vi "Initialise devices.vi"() -> (5 "Number of connected devices":u32, 6 "Device handles":u32[](array[numeric]), 7 "Laser comms. error":errorcluster[](array[cluster]), 8 "Get lasers serial num. error":errorcluster, 9 "Device detection error":errorcluster, 10 "Device initialisation errors":errorcluster[](array[cluster]))   [LabVIEW 2014]
uses:
  Commands.ctl
  Coherent global.vi
panel:
  # "PN 05/11/2014"
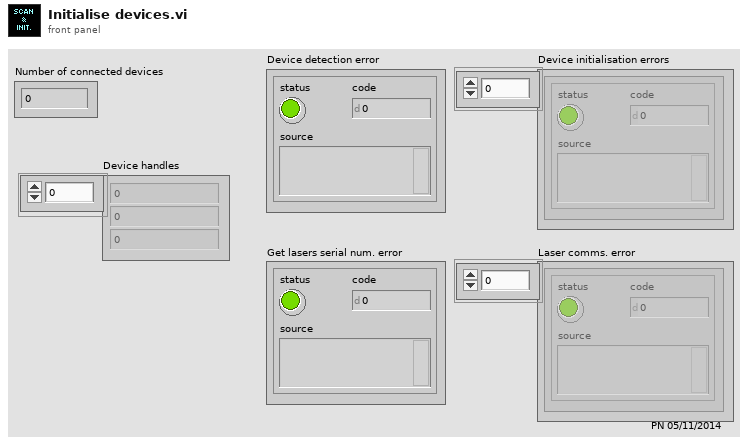
[diagram p1: front panel]
types:
  T1 = typedef "Commands.ctl" = u8
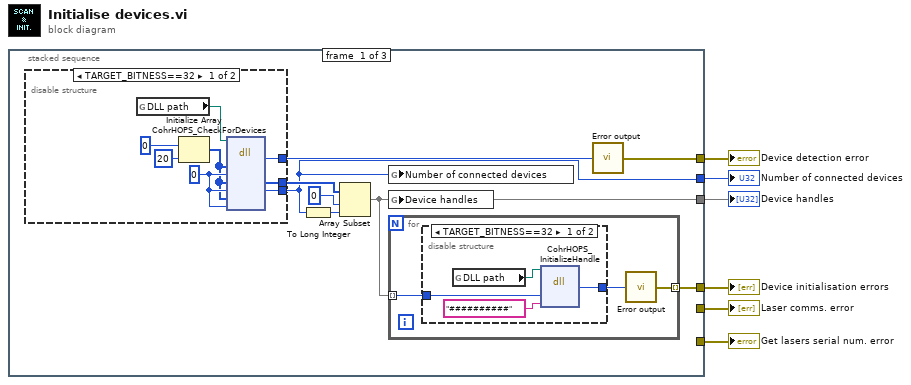
[diagram p0: block diagram]
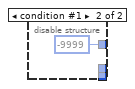
[diagram p2: hidden frame]
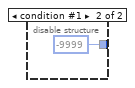
[diagram p3: hidden frame]
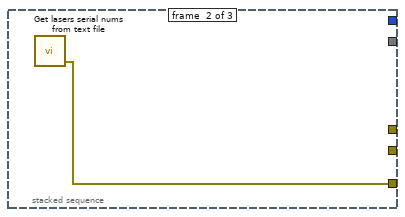
[diagram p4: hidden frame]
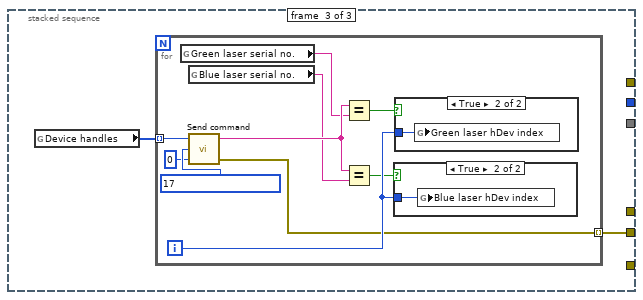
[diagram p5: hidden frame]
diagram:
  n1 = stacked-sequence {
    tunnel: [w11 _ _] -> w6
    tunnel: [w10 _ _] -> w5
    tunnel: [w9 _ _] -> w4
    tunnel: [w7 _ _] -> w3
    tunnel: [_ w32 _] -> w2
    tunnel: [_ _ w33] -> w1
    frame #0 {
      n2 = disable-structure shown="TARGET_BITNESS==32" {
        disable-tunnel: [w18 -9999 ("return value")] -> w12
        disable-tunnel: [w17 _] -> w8
        disable-tunnel: [w16 _] -> w7
        frame condition #0 (active) {
          w22 = u32 0 ("Input Value")
          n3 = global read "Coherent global.vi" "DLL path"() -> (w15:path)
          n4 = Initialize Array(u32 0 ("Input Value"), 20 ("dimension size")) -> (w19:u32[])
          n5 = dll-call lib="C:/Program Files (x86)/Coherent/HOPS/CohrHOPS.dll" fn="CohrHOPS_CheckForDevices"(path in=w15, "devicesConnected"=w19, "numberOfDevicesConnected"=w22, "devicesAdded"=w19, "numberOfDevicesAdded"=w22, "devicesRemoved"=w19, "numberOfDevicesRemoved"=w22) -> ("return value"=w18:i32, "devicesAdded"=w17:u32[], "numberOfDevicesAdded"=w16:u32)  [unwired: 6 in, 2 out]
        }
        frame condition #1 {
        }
      }
      n6 = To Long Integer(number=w7) -> (32bit integer=w14:i32)
      n7 = Array Subset(array=w8, index=0, length=w14) -> (w11:u32[])
      n8 = global write "Coherent global.vi" "Number of connected devices"(w7) -> ()
      n9 = global write "Coherent global.vi" "Device handles"(w11) -> ()
      n10 = for {
        tunnel: w11 -> [w26] mode=indexing
        tunnel: [w24] -> w9 mode=indexing
        n11 = disable-structure shown="TARGET_BITNESS==32" {
          disable-tunnel: w26 -> [w30 _]
          disable-tunnel: [w29 -9999 ("return value")] -> w25
          frame condition #0 (active) {
            n12 = global read "Coherent global.vi" "DLL path"() -> (w27:path)
            n13 = dll-call lib="C:/Program Files (x86)/Coherent/HOPS/CohrHOPS.dll" fn="CohrHOPS_InitializeHandle"(path in=w27, "handle"=w30, "headType"="##########") -> ("return value"=w29:i32)  [unwired: 4 in, 2 out]
          }
          frame condition #1 {
          }
        }
        n14 = call "Error output.vi"("I32 err code"=w25) -> ("Error Out"=w24:errorcluster)
      }
      n15 = call "Error output.vi"("I32 err code"=w12) -> ("Error Out"=w10:errorcluster)
    }
    frame #1 {
      n16 = call "Get lasers serial nums from text file.vi"() -> ("Error"=w32:errorcluster)  [unwired: 2 in, 2 out]
    }
    frame #2 {
      n17 = global read "Coherent global.vi" "Device handles"() -> (w34:u32[])
      n18 = for {
        tunnel: w34 -> [w43] mode=indexing
        tunnel: [w41] -> w33 mode=indexing
        i -> [w44]
        n19 = global read "Coherent global.vi" "Green laser serial no."() -> (w38:string)
        n20 = global read "Coherent global.vi" "Blue laser serial no."() -> (w39:string)
        n21 = call "Send command.vi"("Value"=u16 0, "Command"=T1 17, "Device handle"=w43) -> ("Error"=w41:errorcluster, "response"=w40:string)  [unwired: 1 out]
        n22 = Equal?(x=w40, y=w38) -> (x = y?=w37:bool)
        n23 = Equal?(x=w40, y=w39) -> (x = y?=w36:bool)
        n24 = case shown="True" w36 {
          tunnel: w44 -> [_ w46]
          frame False {
          }
          frame True {
            n25 = global write "Coherent global.vi" "Blue laser hDev index"(w46) -> ()
          }
        }
        n26 = case shown="True" w37 {
          tunnel: w44 -> [_ w45]
          frame False {
          }
          frame True {
            n27 = global write "Coherent global.vi" "Green laser hDev index"(w45) -> ()
          }
        }
      }
    }
  }
  "Device handles" <- w6
  "Device detection error" <- w5
  "Device initialisation errors" <- w4
  "Number of connected devices" <- w3
  "Get lasers serial num. error" <- w2
  "Laser comms. error" <- w1
